vi "updateDisplay.vi"(8 "error in (no error)":errorcluster, 11 "ActionEditor in":refnum<class "ActionEditor.lvclass">) -> (0 "error out":errorcluster, 3 "ActionEditor out":refnum<class "ActionEditor.lvclass">)   [LabVIEW 2011, in "Views.lvlib" / "ScriptEditor.lvlib" / "ActionEditor.lvclass"]
uses:
  ActionEditor.lvclass
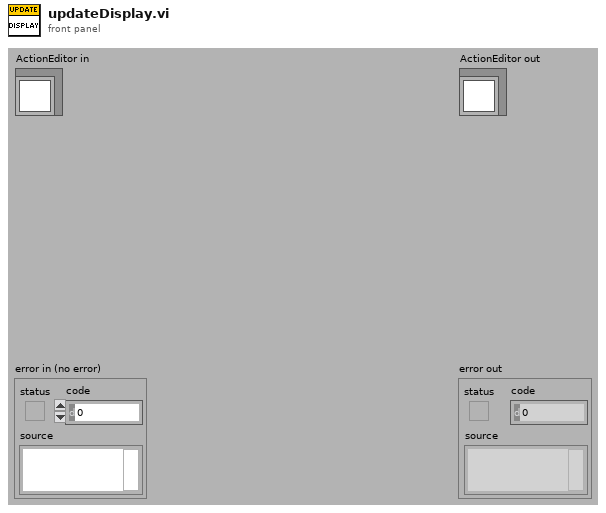
[diagram p1: front panel]
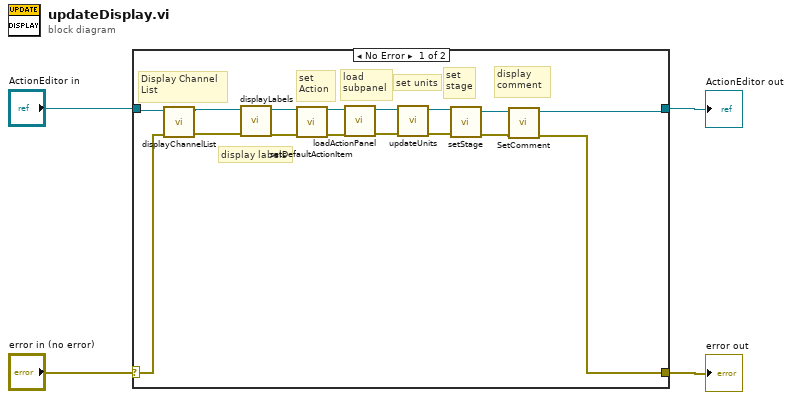
[diagram p0: block diagram]
diagram:
  n1 = case shown="No Error" "error in (no error)" {
    selector: "error in (no error)" -> [w17 w22]
    tunnel: [w13 w22] -> w3
    tunnel: [w14 w21] -> w1
    tunnel: "ActionEditor in" -> [w18 w21]
    frame No Error {
      # "display labels"
      # "set units"
      # "load\nsubpanel"
      # "display \ncomment"
      # "set\nstage"
      # "set\nAction"
      # "Display Channel\nList"
      n2 = call "displayChannelList.vi"("error in (no error)"=w17, "ActionEditor in"=w18) -> ("error out"=w7:errorcluster, "ActionEditor out"=w8:refnum<class "ActionEditor.lvclass">)  [unwired: 8 in]
      n3 = call "displayLabels.vi"("error in (no error)"=w7, "ActionEditor in"=w8) -> ("error out"=w5:errorcluster, "ActionEditor out"=w6:refnum<class "ActionEditor.lvclass">)  [unwired: 8 in]
      n4 = call "setDefaultActionItem.vi"("error in (no error)"=w5, "ActionEditor in"=w6) -> ("error out"=w15:errorcluster, "ActionEditor out"=w16:refnum<class "ActionEditor.lvclass">)  [unwired: 8 in]
      n5 = call "loadActionPanel.vi"("error in (no error)"=w15, "ActionEditor in"=w16) -> ("error out"=w10:errorcluster, "ActionEditor out"=w12:refnum<class "ActionEditor.lvclass">)  [unwired: 8 in]
      n6 = call "updateUnits.vi"("error in (no error)"=w10, "ActionEditor in"=w12) -> ("error out"=w9:errorcluster, "ActionEditor out"=w11:refnum<class "ActionEditor.lvclass">)  [unwired: 8 in]
      n7 = call "setStage.vi"("error in (no error)"=w9, "ActionEditor in"=w11) -> ("error out"=w19:errorcluster, "ActionEditor out"=w20:refnum<class "ActionEditor.lvclass">)  [unwired: 8 in]
      n8 = call "SetComment.vi"("error in (no error)"=w19, "ActionEditor in"=w20) -> ("error out"=w13:errorcluster, "ActionEditor out"=w14:refnum<class "ActionEditor.lvclass">)  [unwired: 8 in]
    }
    frame Error {
    }
  }
  "error out" <- w3
  "ActionEditor out" <- w1
